vi "To 1D Int Tree Data.vi"(10 "1D Int":i64[](array[numeric])) -> (3 "1D Int Tree Data":refnum<class "1D Int.lvclass">)   [LabVIEW 2020, in "NI_VIAnCFGDataStructure.lvlib" / "1D Int.lvclass"]
doc: "Convert an 1D Integer value to Tree Data type."
uses:
  <vilib>/addons/analyzer/VIAnCFGDataStructure/Data Types/Int Array/1D Int.lvclass
  <vilib>/addons/analyzer/VIAnCFGDataStructure/Data Types/Int Array/1D Int.lvclass/1D Int.ctl
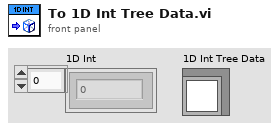
[diagram p1: front panel]
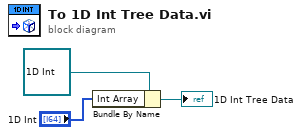
[diagram p0: block diagram]
diagram:
  n1 = Bundle By Name(cluster=refnum<class "1D Int.lvclass"> refnum ("Int Array.lvclass"), "Int Array"="1D Int") -> (→"1D Int Tree Data":refnum<class "1D Int.lvclass">)
